vi "16 JSON Packets.vi"() -> ()   [LabVIEW 2020]
uses:
  _Subs/OpenDiagram/Open_XControl.xctl
panel:
  out "Class B Grade element":cluster{"Name":string, "Grade":i32}={"Name"="Bill", "Grade"=5}
  out "More options":T1={"String"="a string", "Number"=3.14, "Integer"=3, "Friends"=["Fred", "Sally", "Edward", "Kim"]}
  out "Cluster back":cluster{"STRING":string}={"STRING"="a string"}
  out "Complicated":string="{\"Name\":\"Chris\",\"Class A\":{\"Name\":\"EN1\",\"Grades\":[3,4,5]},\"Class B\":{\"Name\":\"EN1\",\"Grades\":[{\"Name\":\"Bill\",\"Grade\":5},{\"Name\":\"Sally\",\"Grade\":3},{\"Name\":\"Kim\",\"Grade\":9}]}}"
  out "More options":string="{\"String\":\"a string\",\"Number\":3.1400000000000001243,\"Integer\":3,\"Friends\":[\"Fred\",\"Sally\",\"Edward\",\"Kim\"]}"
  out "Simple JSON String":string="{\"STRING\":\"a string\"}"
  in  "OpenDiag":refnum<vi>(xcontrol)
  # "16 JSON\nThis code shows a number of tricks for reading JSON Ackets\n\nInstructions:\n1. Hit run to see the constants made into JSON strings and back to clusters again\n2. Try changing the values in the diagram and running again\n3. Try getting different elements from the Cluster that is returned"
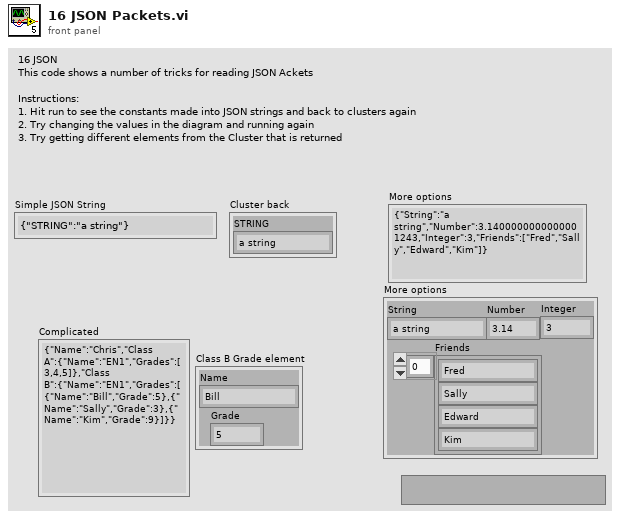
[diagram p1: front panel]
types:
  T1 = cluster{"String":string, "Number":dbl, "Integer":i32, "Friends":string[]}
  T2 = cluster{"Name":string, "Class A":cluster{"Name":string, "Grades":i32[]}, "Class B":cluster{"Name":string, "Grades":cluster{"Name":string, "Grade":i32}[]}}
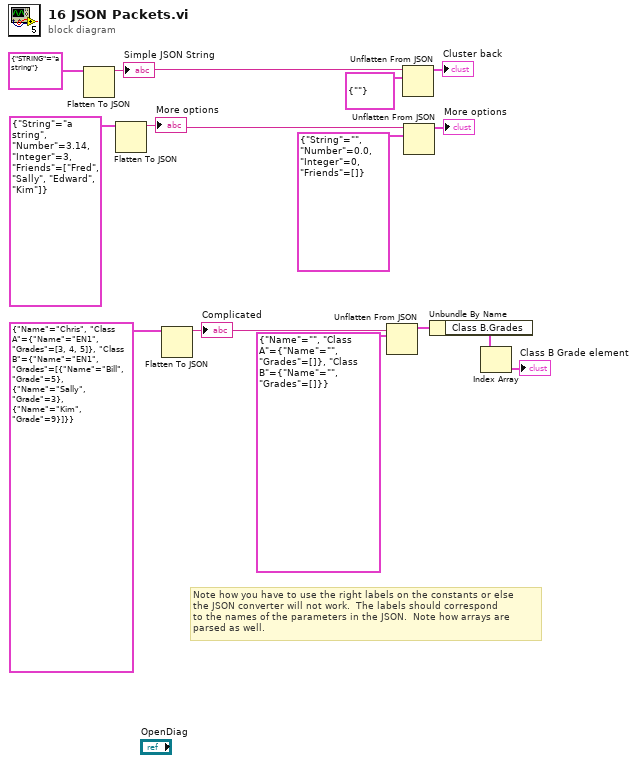
[diagram p0: block diagram]
diagram:
  # "Note how you have to use the right labels on the constants or else\nthe JSON converter will not work.  The labels should correspond\nto the names of the parameters in the JSON.  Note how arrays are\nparsed as well."
  n1 = Flatten To JSON(anything=cluster{"STRING":string} {"STRING"="a string"}) -> (JSON string=w10:string)  [unwired: 2 in, 1 out]
  "Simple JSON String" <- w10
  n2 = Flatten To JSON(anything=T1 {"String"="a string", "Number"=3.14, "Integer"=3, "Friends"=["Fred", "Sally", "Edward", "Kim"]}) -> (JSON string=w8:string)  [unwired: 2 in, 1 out]
  "More options" <- w8
  n3 = Flatten To JSON(anything=T2 {"Name"="Chris", "Class A"={"Name"="EN1", "Grades"=[3, 4, 5]}, "Class B"={"Name"="EN1", "Grades"=[{"Name"="Bill", "Grade"=5}, {"Name"="Sally", "Grade"=3}, {"Name"="Kim", "Grade"=9}]}}) -> (JSON string=w5:string)  [unwired: 2 in, 1 out]
  "Complicated" <- w5
  n4 = Unflatten From JSON(JSON string=w5, type and defaults=T2 {"Name"="", "Class A"={"Name"="", "Grades"=[]}, "Class B"={"Name"="", "Grades"=[]}}) -> (value=w3:T2)  [unwired: 5 in, 1 out]
  n5 = Unflatten From JSON(JSON string=w10, type and defaults=cluster{"STRING":string} {"STRING"=""}) -> (value=→"Cluster back":cluster{"STRING":string})  [unwired: 5 in, 1 out]
  n6 = Unflatten From JSON(JSON string=w8, type and defaults=T1 {"String"="", "Number"=0.0, "Integer"=0, "Friends"=[]}) -> (value=→"More options":T1)  [unwired: 5 in, 1 out]
  n7 = Unbundle By Name(w3) -> ("Class B.Grades"=w2:cluster{"Name":string, "Grade":i32}[])
  n8 = Index Array(array=w2) -> (element=→"Class B Grade element":cluster{"Name":string, "Grade":i32})  [unwired: 1 in]
